vi "Sliders Control.vi"() -> ()   [LabVIEW 2013]
uses:
  Controls/Gripper Status.ctl
  Controls/Finger Status.ctl
  Class/Robotiq.lvclass
  Controls/Gripper Command.ctl
  Controls/Finger Command.ctl
panel:
  out "Gripper Status":T1
  in  "Close":u8(slide) scale=0.0..255.0
  in  "Rate (ms)":u32=10
  in  "Scissor":u8(slide)=100 scale=0.0..255.0
  in  "stop":bool
  in  "Port":u16=502
  in  "IP Address":string="138.100.76.56"
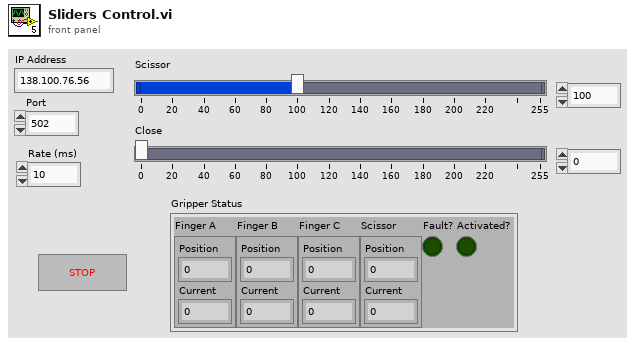
[diagram p1: front panel]
types:
  T1 = typedef "Gripper Status.ctl" = cluster{"Finger A":T2, "Finger B":T2, "Finger C":T2, "Scissor":T2, "Fault?":bool, "Activated?":bool}
  T2 = typedef "Finger Status.ctl" = cluster{"Position":dbl, "Current":dbl}
  T3 = typedef "Gripper Command.ctl" = cluster{"Finger A":T4, "Finger B":T4, "Finger C":T4, "Scissor":T4}
  T4 = typedef "Finger Command.ctl" = cluster{"Position":u8, "Speed":u8, "Force":u8}
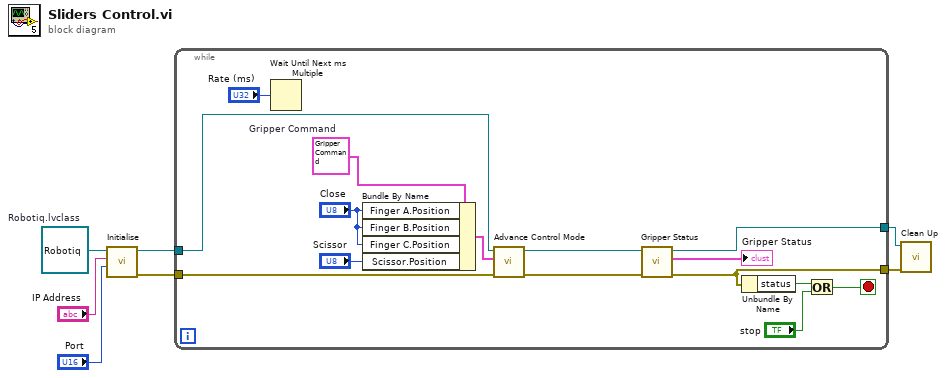
[diagram p0: block diagram]
diagram:
  w5 = refnum<class "Robotiq.lvclass"> refnum  # Robotiq.lvclass
  n1 = call "Initialise.vi"("Port"="Port", "IP Address"="IP Address", "Robotiq in"=w5) -> ("error out"=w3:errorcluster, "Robotiq out"=w4:refnum<class "Robotiq.lvclass">)  [unwired: 7 in]
  n2 = while {
    tunnel: w3 -> [w18]
    tunnel: [w9] -> w1
    tunnel: w4 -> [w19]
    tunnel: [w10] -> w2
    stop <- w20 stop-if-true
    w16 = T3 {"Finger A"={"Position"=0, "Speed"=255, "Force"=255}, "Finger B"={"Position"=0, "Speed"=255, "Force"=255}, "Finger C"={"Position"=0, "Speed"=255, "Force"=255}, "Scissor"={"Position"=0, "Speed"=255, "Force"=255}}  # Gripper Command
    n3 = Wait Until Next ms Multiple(millisecond multiple="Rate (ms)") -> ()  [unwired: 1 out]
    n4 = Bundle By Name(cluster=w16, "Finger A.Position"="Close", "Finger B.Position"="Close", "Finger C.Position"="Close", "Scissor.Position"="Scissor") -> (w13:T3)
    n5 = call "Advance Control Mode.vi"("error in (no error)"=w18, "Gripper Command"=w13, "Robotiq in"=w19) -> ("error out"=w11:errorcluster, "Robotiq out"=w12:refnum<class "Robotiq.lvclass">)  [unwired: 7 in]
    n6 = call "Gripper Status.vi"("error in (no error)"=w11, "Robotiq in"=w12) -> ("error out"=w9:errorcluster, "Gripper Status"=→"Gripper Status":T1, "Robotiq out"=w10:refnum<class "Robotiq.lvclass">)  [unwired: 7 in]
    n7 = Unbundle By Name(w9) -> ("status"=w22:bool)
    n8 = Or(x=w22, y="stop") -> (x .or. y?=w20:bool)
  }
  n9 = call "Clean Up.vi"("error in (no error)"=w1, "Robotiq in"=w2) -> ()  [unwired: 8 in, 2 out]
